vi "feedback_run.vi"   [LabVIEW 2019]
uses:
  lib/libSimulationControl/libSimulationControl.lvlib
  lib/libFileFunctions/libFileFunctions.lvlib
panel:
  # "*******************************************************************\nBiogas Plant Control\n\nAuthor: Paul Zügel\nGCSC-Frankfurt am Main 2020\n\n*******************************************************************"
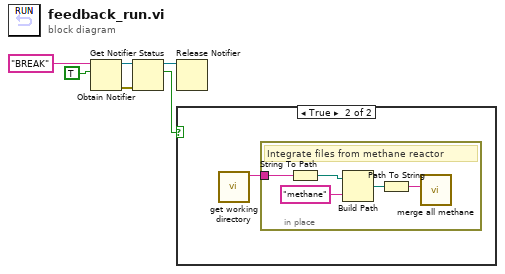
[diagram p0: block diagram]
diagram:
  n1 = Obtain Notifier(name (unnamed)="BREAK", notification data type=TRUE) -> (notifier out=w4:refnum<notifier>, error out=w3:errorcluster)  [unwired: 2 in, 1 out]
  n2 = Get Notifier Status(notifier=w4, error in (no error)=w3) -> (notifier out=w1:refnum<notifier>, current notification=w2:bool)  [unwired: 3 out]
  n3 = Release Notifier(notifier=w1) -> ()  [unwired: 2 in, 3 out]
  n4 = case shown="True" w2 {
    frame False {
    }
    frame True {
      n5 = call "get working directory.vi"() -> ("function return"=w7:string)  [unwired: 10 in, 1 out]
      n6 = in-place {
        in-place-border: w7 -> [w12]
        # "Integrate files from methane reactor"
        n7 = String To Path(string=w12) -> (path=w11:path)
        n8 = Build Path(base path=w11, name or relative path="methane") -> (appended path=w9:path)
        n9 = Path To String(path=w9) -> (string=w8:string)
        n10 = call "merge all methane.vi"("methane_dir"=w8) -> ()  [unwired: 10 in, 1 out]
      }
    }
  }
